vi "AlliGator Load Single Gate Image from HDF5 v 0.6b.vi"(6 "Action":T1, 8 "error in (no error)":errorcluster, 10 "File Info":variant, 11 "Gate Index":i32) -> (0 "error out":errorcluster, 1 "Data 2":sgl[][](array[numeric]), 3 "Data 1":sgl[][](array[numeric]))   [LabVIEW 2021, in "AlliGator HDF5.lvlib"]
doc: "Loads single gate image (or dual-channel images) from HDF5 FLI dataset file (v0.6b)."
uses:
  AlliGator HDF5.lvlib
  AlliGator FLI Image Stack Action.ctl
  AlliGator HDF5 FLI File Loading Information v0.6.ctl
  <vilib>/addons/h5labview2/base/lib_path.vi
  <vilib>/addons/h5labview2/base/H5Equery.vi
  <vilib>/Utility/error.llb/Error Cluster From Error Code.vi
  <vilib>/addons/h5labview2/base/hid_t.ctl
  <vilib>/addons/h5labview2/dataset/H5Dread.llb/H5Dread.xnode
  <vilib>/ErrorRing/Error Ring.xnode
  <vilib>/addons/h5labview2/file/H5F.lvlib
  <vilib>/addons/h5labview2/group/H5G.lvlib
  AlliGator Dual-Channel Datasets.lvlib
panel:
  # "see the AlliGator License on the block diagram (Ctrl+E or Window:Show Block Diagram)"
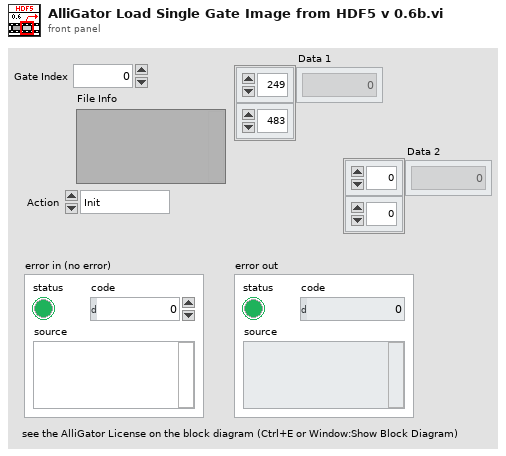
[diagram p1: front panel]
types:
  T1 = typedef "AlliGator HDF5.lvlib/AlliGator FLI Image Stack Action.ctl" = enum16{"Init", "Get Image", "Close"}
  T2 = typedef "AlliGator HDF5.lvlib/AlliGator HDF5 FLI File Loading Information v0.6.ctl" = cluster{"HDF5 File Path":path, "Data Type":string, "# Datasets in Series":i32, "Dataset ID in Series":i32, "Channel Names":string[]}
  T3 = typedef "hid_t.ctl" = i64
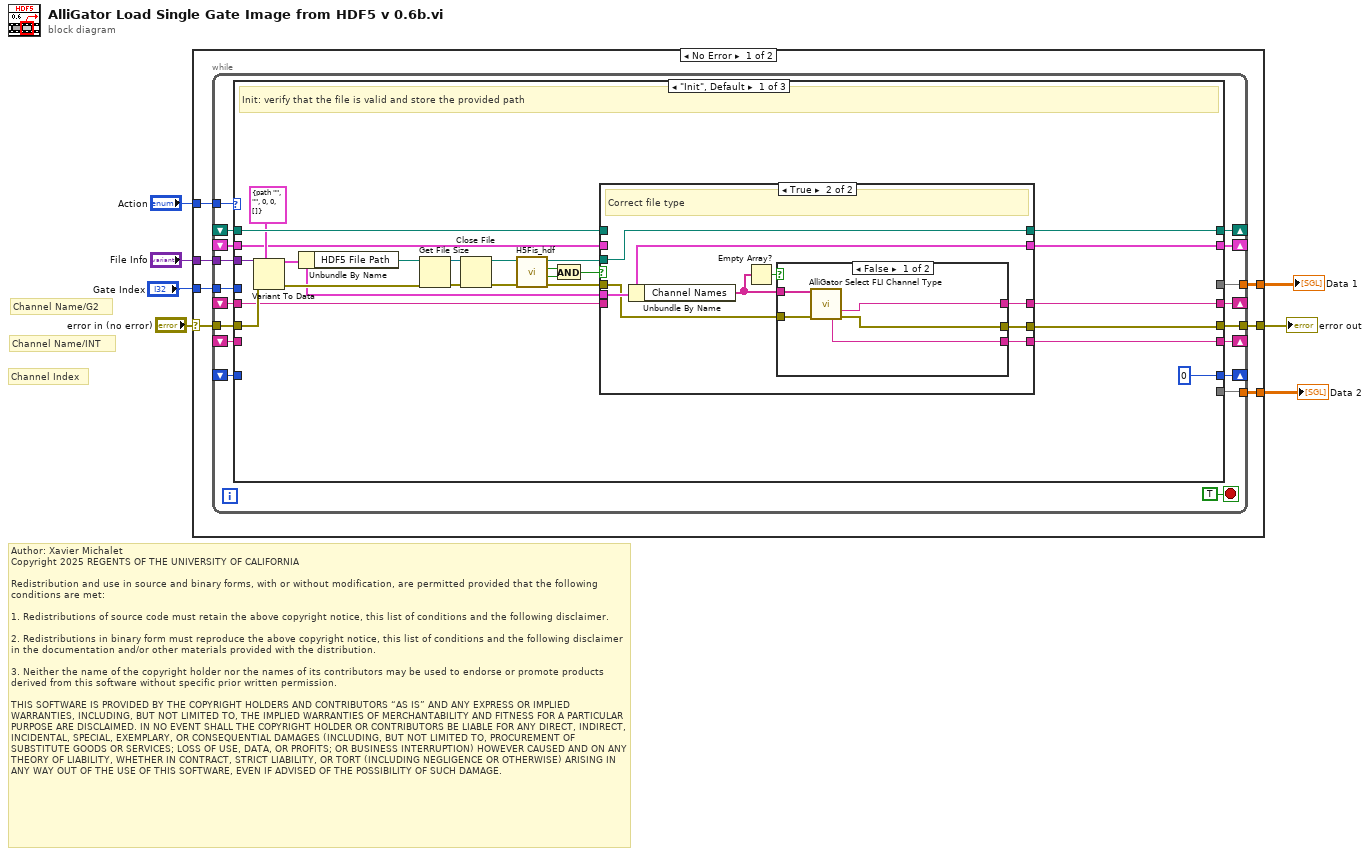
[diagram p0: block diagram]
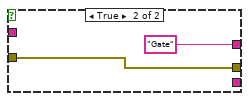
[diagram p3: hidden frame]
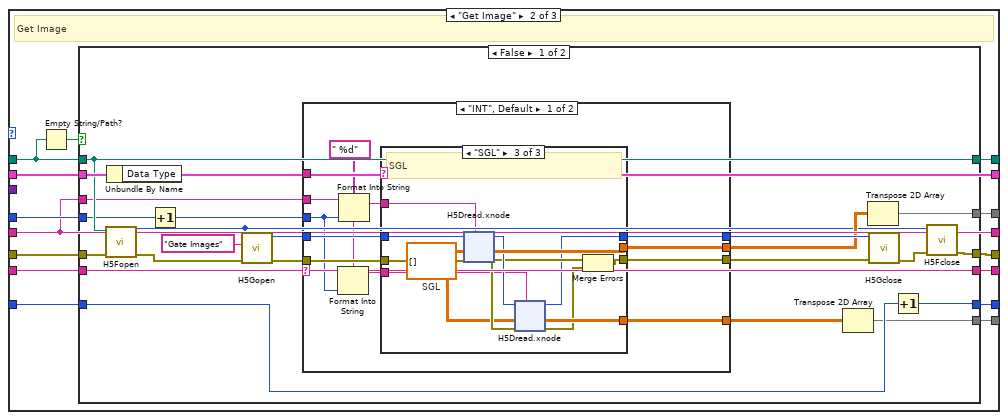
[diagram p4: hidden frame]
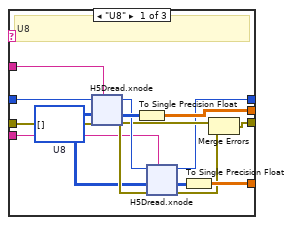
[diagram p5: hidden frame]
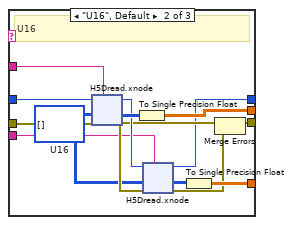
[diagram p6: hidden frame]
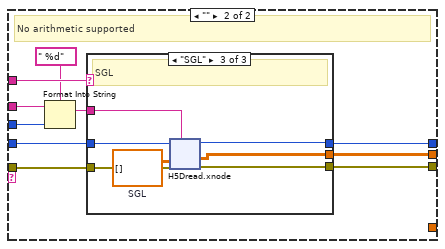
[diagram p7: hidden frame]
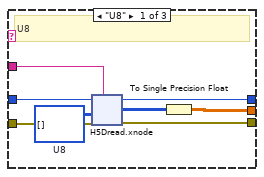
[diagram p8: hidden frame]
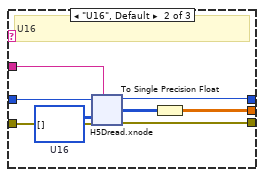
[diagram p9: hidden frame]
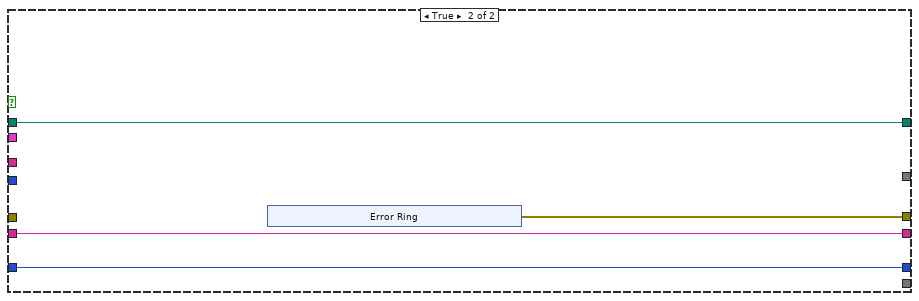
[diagram p10: hidden frame]
diagram:
  # "Author: Xavier Michalet\nCopyright 2025 REGENTS OF THE UNIVERSITY OF CALIFORNIA\n\nRedistribution and use in source and binary forms, with or without modification, are permitted provided that the following conditions are met:\n\n1. Redistributions of source code must retain the above copyright notice, this list of conditions and the following disclaimer.\n\n2. Redistributions in binary form must reproduce the above copyright notice, this list of conditions and the following disclaimer in the documentation and/or other materials provided with the distribution.\n\n3. Neither the name of the copyright holder nor the names of its contributors may be used to endorse or promote products derived from this software without specific prior written permission.\n\nTHIS SOFTWARE IS PROVIDED BY THE COPYRIGHT HOLDERS AND CONTRIBUTORS “AS IS” AND ANY EXPRESS OR IMPLIED WARRANTIES, INCLUDING, BUT NOT LIMITED TO, THE IMPLIED WARRANTIES OF MERCHANTABILITY AND FITNESS FOR A PARTICULAR PURPOSE ARE DISCLAIMED. IN NO EVENT SHALL THE COPYRIGHT HOLDER OR CONTRIBUTORS BE LIABLE FOR ANY DIRECT, INDIRECT, INCIDENTAL, SPECIAL, EXEMPLARY, OR CONSEQUENTIAL DAMAGES (INCLUDING, BUT NOT LIMITED TO, PROCUREMENT OF SUBSTITUTE GOODS OR SERVICES; LOSS OF USE, DATA, OR PROFITS; OR BUSINESS INTERRUPTION) HOWEVER CAUSED AND ON ANY THEORY OF LIABILITY, WHETHER IN CONTRACT, STRICT LIABILITY, OR TORT (INCLUDING NEGLIGENCE OR OTHERWISE) ARISING IN ANY WAY OUT OF THE USE OF THIS SOFTWARE, EVEN IF ADVISED OF THE POSSIBILITY OF SUCH DAMAGE."
  # "Channel Index"
  # "Channel Name/INT"
  # "Channel Name/G2"
  n1 = case shown="No Error" "error in (no error)" {
    selector: "error in (no error)" -> [w13 w343]
    tunnel: [w12 w343] -> w6
    tunnel: "Action" -> [w14 _]
    tunnel: "File Info" -> [w11 _]
    tunnel: "Gate Index" -> [w10 _]
    tunnel: [w9 _] -> w2
    tunnel: [w8 _] -> w1
    frame No Error {
      n2 = while {
        tunnel: w14 -> [w31]
        tunnel: w13 -> [w30]
        tunnel: [w29] -> w12
        tunnel: w11 -> [w28]
        shift-right: [w27] -> _
        shift-left: _ -> [w26]
        tunnel: w10 -> [w25]
        tunnel: [w24] -> w9
        shift-right: [w23] -> _
        shift-left: _ -> [w22]
        shift-right: [w21] -> _
        shift-left: _ -> [w20]
        shift-right: [w19] -> _
        shift-left: _ -> [w18]
        shift-right: [w17] -> _
        shift-left: _ -> [w16]
        tunnel: [w15] -> w8
        stop <- TRUE stop-if-true
        n3 = case shown="\"Init\", Default" w31 {
          tunnel: w30 -> [w43 w85 w342]
          tunnel: [w45 w88 w342] -> w29
          tunnel: w28 -> [w44 _ _]
          tunnel: [w47 w89 _] -> w27
          tunnel: w26 -> [w46 w87 _]
          tunnel: w25 -> [_ w84 _]
          tunnel: [_ w83 _] -> w24
          tunnel: [w39 w82 _] -> w23
          tunnel: w22 -> [w38 w82 _]
          tunnel: [w36 w81 _] -> w21
          tunnel: w20 -> [w35 w81 _]
          tunnel: [w34 w79 _] -> w19
          tunnel: w18 -> [_ w80 _]
          tunnel: [0 w76 _] -> w17
          tunnel: w16 -> [_ w78 _]
          tunnel: [_ w77 _] -> w15
          frame "Init", Default {
            # "Init: verify that the file is valid and store the provided path"
            n4 = Variant To Data(error in=w43, type=T2 {"HDF5 File Path"=path "", "Data Type"="", "# Datasets in Series"=0, "Dataset ID in Series"=0, "Channel Names"=[]} ("HDF5 FLI File Loading Information"), Variant=w44) -> (data=w37:T2, error out=w41:errorcluster)
            n5 = Unbundle By Name(w37) -> ("HDF5 File Path"=w40:path)
            n6 = Get File Size(file=w40, error in=w41) -> (refnum out=w53:refnum<file>, 0:w54:errorcluster)  [unwired: 1 out]
            n7 = Close File(refnum=w53, error in=w54) -> (path=w52:path, error out=w51:errorcluster)
            n8 = call <vilib>:"H5Fis_hdf.vi"("error in (no error)"=w51, "path in"=w52) -> ("error out"=w49:errorcluster, "valid?"=w55:bool, "exists?"=w56:bool, "path out"=w48:path)  [unwired: 6 in]
            n9 = And(x=w56, y=w55) -> (x .and. y?=w50:bool)
            n10 = case shown="True" w50 {
              tunnel: w49 -> [w59 w63]
              tunnel: w48 -> [_ w68]
              tunnel: [w60 w68] -> w47
              tunnel: w46 -> [w60 _]
              tunnel: [w59 w62] -> w45
              tunnel: [w58 w67] -> w39
              tunnel: w38 -> [w58 _]
              tunnel: w37 -> [_ w67]
              tunnel: [w57 w65] -> w36
              tunnel: w35 -> [w57 _]
              tunnel: [_ w61] -> w34
              frame False {
                # "not legible"
              }
              frame True {
                # "Correct file type"
                n11 = Unbundle By Name(w67) -> ("Channel Names"=w64:string[])
                n12 = Empty Array?(array=w64) -> (empty?=w66:bool)
                n13 = case shown="False" w66 {
                  tunnel: [w71 "Gate" ("Gate Names")] -> w65
                  tunnel: w64 -> [w69 _]
                  tunnel: w63 -> [w73 w75]
                  tunnel: [w72 w75] -> w62
                  tunnel: [w70 _] -> w61
                  frame False {
                    n14 = call "AlliGator Select FLI Channel Type.vi"("Available Channel Names"=w69, "error in (no error)"=w73) -> ("G2 Channel Name (or single Gate Name)"=w71:string, "INT Channel Name (or empty)"=w70:string, "error out"=w72:errorcluster)  [unwired: 5 in, 6 out]
                  }
                  frame True {
                  }
                }
              }
            }
          }
          frame "Get Image" {
            # "Get Image"
            n15 = Empty String/Path?(string/path=w87) -> (empty?=w86:bool)
            n16 = case shown="False" w86 {
              tunnel: [w107 w337] -> w89
              tunnel: w87 -> [w107 w337]
              tunnel: [w109 w336] -> w88
              tunnel: w85 -> [w108 _]
              tunnel: w84 -> [w106 _]
              tunnel: [w101 _] -> w83
              tunnel: w82 -> [w100 _]
              tunnel: w81 -> [w95 _]
              tunnel: w80 -> [w94 w335]
              tunnel: [w94 w335] -> w79
              tunnel: w78 -> [w92 w334]
              tunnel: [w90 _] -> w77
              tunnel: [w91 w334] -> w76
              frame False {
                n17 = call <vilib>:"H5Fopen.vi"("error in (no error)"=w108, "path"=w107) -> ("error out"=w112:errorcluster, "ref out"=w96:T3)  [unwired: 8 in]
                n18 = Unbundle By Name(w100) -> ("Data Type"=w99:string)
                n19 = Increment(x=w106) -> (x+1=w105:i32)
                n20 = call <vilib>:"H5Gopen.vi"("error in (no error)"=w112, "name"="Gate Images", "ref in"=w96) -> ("error out"=w98:errorcluster, "group out"=w97:T3)  [unwired: 7 in]
                n21 = case shown="\"INT\", Default" w94 {
                  selector: w94 -> [w118 _]
                  tunnel: [w125 w265] -> w104
                  tunnel: [w123 w263] -> w102
                  tunnel: w99 -> [w122 w262]
                  tunnel: w98 -> [w121 w261]
                  tunnel: w97 -> [w120 w260]
                  tunnel: w95 -> [w119 w259]
                  tunnel: w105 -> [w116 w257]
                  tunnel: [w114 w256] -> w103
                  tunnel: [w113 _] -> w93
                  frame "INT", Default {
                    w117 = " %d" ("format string")
                    n22 = Format Into String(format string=w117, initial string=w118, w116) -> (resulting string=w115:string)  [unwired: 1 in, 1 out]
                    n23 = Format Into String(format string=w117, initial string=w119, w116) -> (resulting string=w124:string)  [unwired: 1 in, 1 out]
                    n24 = case shown="\"SGL\"" w122 {
                      tunnel: w120 -> [w139 w183 w225]
                      tunnel: [w132 w176 w219] -> w125
                      tunnel: [w137 w181 w224] -> w114
                      tunnel: w124 -> [w136 w180 w223]
                      tunnel: [w127 w171 w215] -> w123
                      tunnel: w121 -> [w135 w179 w222]
                      tunnel: w115 -> [w128 w172 w216]
                      tunnel: [w129 w173 w217] -> w113
                      frame "U8" {
                        w131 = u8[][] []  # U8
                        # "U8"
                        n25 = xnode "H5Dread.xnode"("dataset name (this)"=w136, "error in (no error)"=w135, "default"=w131, "ref in"=w139) -> ("error out"=w133:errorcluster, "data"=w138:u8[][], "ref out"=w134:T3)  [unwired: 2 in, 1 out]
                        n26 = To Single Precision Float(number=w138) -> (single precision float=w137:sgl[][])
                        n27 = xnode "H5Dread.xnode"("dataset name (this)"=w128, "error in (no error)"=w133, "default"=w131, "ref in"=w134) -> ("error out"=w126:errorcluster, "data"=w130:u8[][], "ref out"=w132:T3)  [unwired: 2 in, 1 out]
                        n28 = To Single Precision Float(number=w130) -> (single precision float=w129:sgl[][])
                        n29 = Merge Errors(w133, w126) -> (w127:errorcluster)
                      }
                      frame "U16", Default {
                        w175 = u16[][] []  # U16
                        # "U16"
                        n30 = xnode "H5Dread.xnode"("dataset name (this)"=w180, "error in (no error)"=w179, "default"=w175, "ref in"=w183) -> ("error out"=w177:errorcluster, "data"=w182:u16[][], "ref out"=w178:T3)  [unwired: 2 in, 1 out]
                        n31 = To Single Precision Float(number=w182) -> (single precision float=w181:sgl[][])
                        n32 = xnode "H5Dread.xnode"("dataset name (this)"=w172, "error in (no error)"=w177, "default"=w175, "ref in"=w178) -> ("error out"=w170:errorcluster, "data"=w174:u16[][], "ref out"=w176:T3)  [unwired: 2 in, 1 out]
                        n33 = To Single Precision Float(number=w174) -> (single precision float=w173:sgl[][])
                        n34 = Merge Errors(w177, w170) -> (w171:errorcluster)
                      }
                      frame "SGL" {
                        w218 = sgl[][] []  # SGL
                        # "SGL"
                        n35 = xnode "H5Dread.xnode"("dataset name (this)"=w223, "error in (no error)"=w222, "default"=w218, "ref in"=w225) -> ("error out"=w220:errorcluster, "data"=w224:sgl[][], "ref out"=w221:T3)  [unwired: 2 in, 1 out]
                        n36 = xnode "H5Dread.xnode"("dataset name (this)"=w216, "error in (no error)"=w220, "default"=w218, "ref in"=w221) -> ("error out"=w214:errorcluster, "data"=w217:sgl[][], "ref out"=w219:T3)  [unwired: 2 in, 1 out]
                        n37 = Merge Errors(w220, w214) -> (w215:errorcluster)
                      }
                    }
                  }
                  frame "" {
                    # "No arithmetic supported"
                    n38 = Format Into String(format string=" %d", initial string=w259, w257) -> (resulting string=w264:string)  [unwired: 1 in, 1 out]
                    n39 = case shown="\"SGL\"" w262 {
                      tunnel: w260 -> [w273 w296 w318]
                      tunnel: [w266 w291 w314] -> w265
                      tunnel: [w271 w294 w317] -> w256
                      tunnel: w264 -> [w270 w293 w316]
                      tunnel: [w268 w290 w313] -> w263
                      tunnel: w261 -> [w269 w292 w315]
                      frame "U8" {
                        w267 = u8[][] []  # U8
                        # "U8"
                        n40 = xnode "H5Dread.xnode"("dataset name (this)"=w270, "error in (no error)"=w269, "default"=w267, "ref in"=w273) -> ("error out"=w268:errorcluster, "data"=w272:u8[][], "ref out"=w266:T3)  [unwired: 2 in, 1 out]
                        n41 = To Single Precision Float(number=w272) -> (single precision float=w271:sgl[][])
                      }
                      frame "U16", Default {
                        w289 = u16[][] []  # U16
                        # "U16"
                        n42 = xnode "H5Dread.xnode"("dataset name (this)"=w293, "error in (no error)"=w292, "default"=w289, "ref in"=w296) -> ("error out"=w290:errorcluster, "data"=w295:u16[][], "ref out"=w291:T3)  [unwired: 2 in, 1 out]
                        n43 = To Single Precision Float(number=w295) -> (single precision float=w294:sgl[][])
                      }
                      frame "SGL" {
                        w312 = sgl[][] []  # SGL
                        # "SGL"
                        n44 = xnode "H5Dread.xnode"("dataset name (this)"=w316, "error in (no error)"=w315, "default"=w312, "ref in"=w318) -> ("error out"=w313:errorcluster, "data"=w317:sgl[][], "ref out"=w314:T3)  [unwired: 2 in, 1 out]
                      }
                    }
                  }
                }
                n45 = Transpose 2D Array(2D array=w93) -> (transposed array=w90:sgl[][])
                n46 = Transpose 2D Array(2D array=w103) -> (transposed array=w101:sgl[][])
                n47 = call <vilib>:"H5Gclose.vi"("error in (no error)"=w102, "group in"=w104) -> ("error out"=w110:errorcluster)  [unwired: 9 in]
                n48 = Increment(x=w92) -> (x+1=w91:i32)
                n49 = call <vilib>:"H5Fclose.vi"("error in (no error)"=w110, "ref"=w96) -> ("error out"=w109:errorcluster)  [unwired: 9 in]
              }
              frame True {
                n50 = xnode "Error Ring"() -> ("error out"=w336:errorcluster)
              }
            }
          }
          frame "Close" {
            # "Close File"
          }
        }
      }
    }
    frame Error {
    }
  }
  "Data 1" <- w2
  "error out" <- w6
  "Data 2" <- w1
